vi "Fetch Config.vi"(7 "UI Device Type":T4, 8 "error in (no error)":errorcluster, 10 "ModelNumber":string, 11 "Database in":refnum<queue>) -> (0 "error out":errorcluster, 2 "Model Details Payload":T1={"Serial Numbers"=[], "Hardware Settings Cluster"={"Sensor ID *"=0, "Target Sample Rate (Hz) *"=1000.0, "Steady-State Duration (s) *"=5, "Allowed Tolerance (%) FS *"=0.5, "Max Settling Timeout (s) *"=5, "Physical Channel"="", "Measurement Role"=enum."Reference"}}, 3 "Database out":refnum<queue>)   [LabVIEW 2026, in "Settings.lvlib"]
uses:
  Settings.lvlib
  support/Architecture/Message Queue/Message Cluster.ctl
  controls/UI/Data Entity.ctl
  controls/Messaging Payloads/MSG FetchConfiguration Payload.ctl
  Acquisition/Instrument Specifications Cluster Configuration.ctl
  controls/UI/Measurement Role.ctl
  controls/Messaging Payloads/Fetch Config Payload.ctl
  support/Architecture/Message Queue/Enqueue Message (Single).vi
  support/Architecture/Message Queue/Message Queue.lvlib
  Acquisition/Acquisition.lvlib
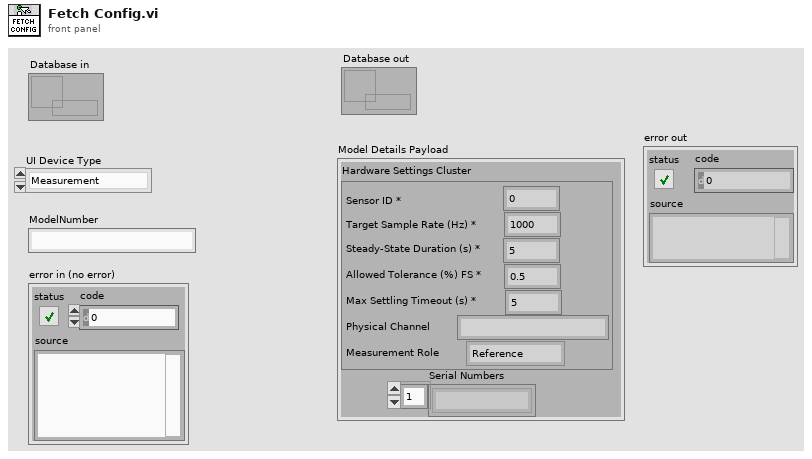
[diagram p1: front panel]
types:
  T1 = typedef "MSG FetchConfiguration Payload.ctl" = cluster{"Serial Numbers":string[], "Hardware Settings Cluster":T2}
  T2 = typedef "Acquisition.lvlib/Instrument Specifications Cluster Configuration.ctl" = cluster{"Sensor ID *":i32, "Target Sample Rate (Hz) *":dbl, "Steady-State Duration (s) *":i32, "Allowed Tolerance (%) FS *":dbl, "Max Settling Timeout (s) *":i32, "Physical Channel":string, "Measurement Role":T3}
  T3 = typedef "Settings.lvlib/Measurement Role.ctl" = enum16{"Reference", "UUT"}
  T4 = typedef "Settings.lvlib/Data Entity.ctl" = enum16{"Measurement", "Controller", " Test Configuration"}
  T5 = typedef "Fetch Config Payload.ctl" = cluster{"Model Number":string, "Notifier":refnum<notifier>, "UI Device Type":T4}
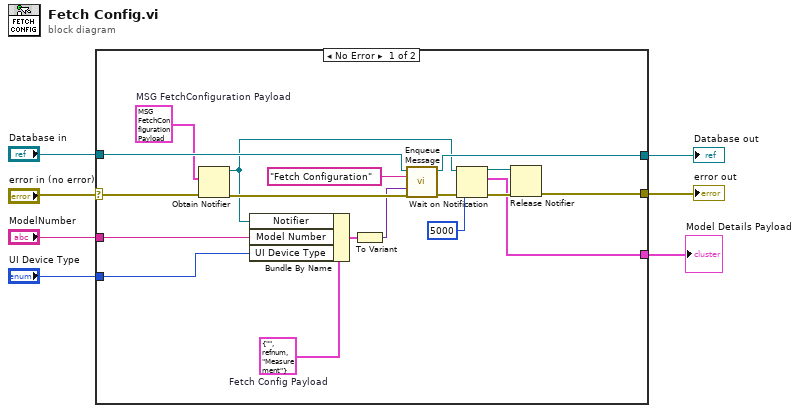
[diagram p0: block diagram]
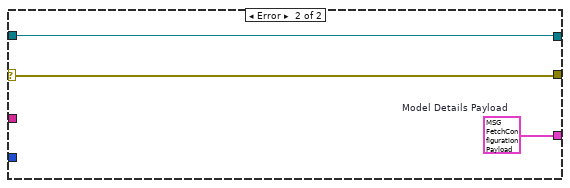
[diagram p2: hidden frame]
diagram:
  n1 = case shown="No Error" "error in (no error)" {
    selector: "error in (no error)" -> [w11 w28]
    tunnel: [w25 w27] -> w7
    tunnel: [w23 w28] -> w6
    tunnel: "Database in" -> [w22 w27]
    tunnel: "ModelNumber" -> [w15 _]
    tunnel: [w9 w26] -> w1
    tunnel: "UI Device Type" -> [w8 _]
    frame No Error {
      w20 = T5 {"Model Number"="", "Notifier"=refnum, "UI Device Type"=enum."Measurement"}  # Fetch Config Payload
      w19 = T1 {"Serial Numbers"=[], "Hardware Settings Cluster"={"Sensor ID *"=0, "Target Sample Rate (Hz) *"=0.0, "Steady-State Duration (s) *"=0, "Allowed Tolerance (%) FS *"=0.0, "Max Settling Timeout (s) *"=5, "Physical Channel"="", "Measurement Role"=enum."Reference"}}  # MSG FetchConfiguration Payload
      n2 = Obtain Notifier(notification data type=w19, error in (no error)=w11) -> (notifier out=w10:refnum<notifier>, error out=w21:errorcluster)  [unwired: 2 in, 1 out]
      n3 = Bundle By Name(cluster=w20, "Notifier"=w10, "Model Number"=w15, "UI Device Type"=w8) -> (w14:T5)
      n4 = To Variant(anything=w14) -> (Variant=w13:variant)
      n5 = call-poly "Enqueue Message.vi"("error in (no error)"=w21, "Message Data"=w13, "Message"="Fetch Configuration", "Message Queue"=w22) -> ("error out"=w16:errorcluster, "dup Message Queue"=w25:refnum<queue>)  [unwired: 6 in]
      n6 = Wait on Notification(notifier=w10, timeout in ms (-1)=5000, error in (no error)=w16) -> (notifier out=w18:refnum<notifier>, notification=w9:T1, error out=w17:errorcluster)  [unwired: 1 in, 1 out]
      n7 = Release Notifier(notifier=w18, error in (no error)=w17) -> (error out=w23:errorcluster)  [unwired: 1 in, 2 out]
    }
    frame Error {
      w26 = T1 {"Serial Numbers"=[], "Hardware Settings Cluster"={"Sensor ID *"=0, "Target Sample Rate (Hz) *"=1000.0, "Steady-State Duration (s) *"=5, "Allowed Tolerance (%) FS *"=0.5, "Max Settling Timeout (s) *"=5, "Physical Channel"="", "Measurement Role"=enum."Reference"}}  # Model Details Payload
    }
  }
  "Database out" <- w7
  "error out" <- w6
  "Model Details Payload" <- w1
